vi "calculationView.vi"(11 "View.lvclass":refnum<class "View.lvclass">) -> ()   [LabVIEW 2016, in "View.lvclass"]
uses:
  View.lvclass
  Controller/Controller.lvclass
  Controller/Controller.lvclass/Controller.ctl
  View.lvclass/View.ctl
panel:
  in  "OK Button":bool
  out "Result":dbl
  in  "secondNumber":dbl
  in  "firstNumber":dbl
  # "+"
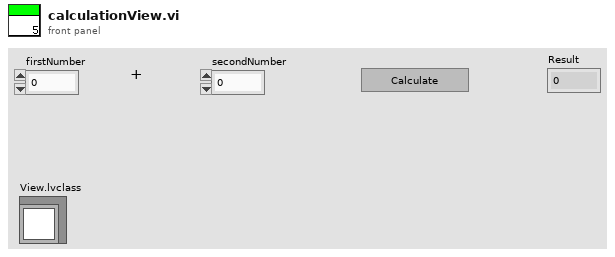
[diagram p1: front panel]
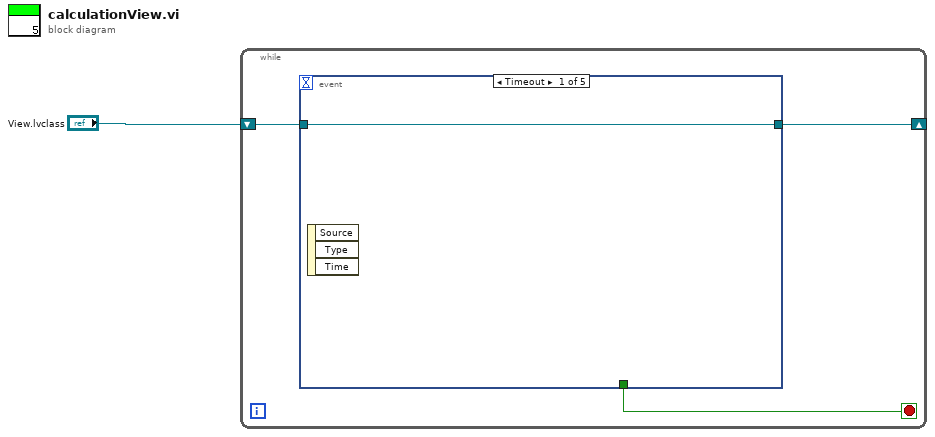
[diagram p0: block diagram]
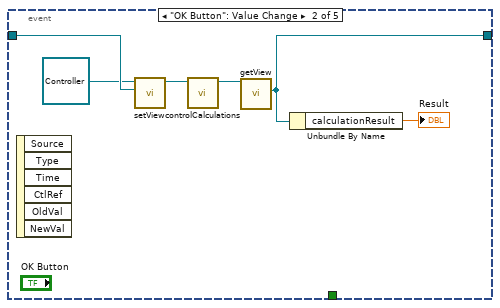
[diagram p2: hidden frame]
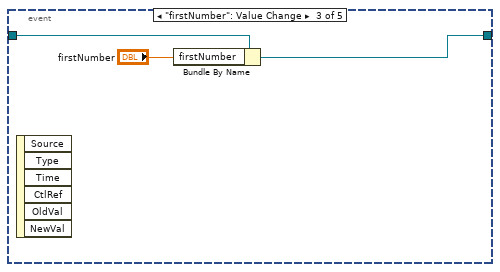
[diagram p3: hidden frame]
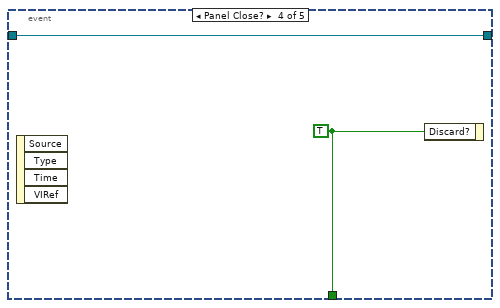
[diagram p4: hidden frame]
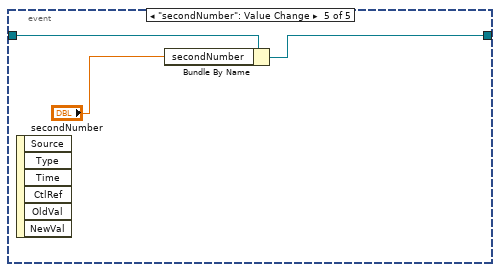
[diagram p5: hidden frame]
diagram:
  n1 = while {
    shift-right: [w2] -> _
    shift-left: "View.lvclass" -> [w4]
    stop <- w3 stop-if-true
    n2 = event shown="[0] Timeout" {
      selector: _ -> [_ _ _ _ _]
      dyn-events: _ -> [_ _ _ _ _]
      timeout: _ -> [_ _ _ _ _]
      tunnel: w4 -> [w5 w10 w14 w15 w18]
      tunnel: [_ _ _ w16 _] -> w3
      tunnel: [w5 w7 w12 w15 w17] -> w2
      event Timeout {
        n3 = event-data() -> ()  [unwired: 1 in, 3 out]
      }
      event "OK Button": Value Change {
        n4 = event-data() -> ()  [unwired: 1 in, 6 out]
        n5 = call "setView.vi"("View.lvclass"=w10, "Controller in"=refnum<class "Controller.lvclass"> refnum) -> ("Controller out"=w11:refnum<class "Controller.lvclass">)  [unwired: 9 in]
        n6 = call "controlCalculations.vi"("Controller In"=w11) -> ("Controller.lvclass"=w9:refnum<class "Controller.lvclass">)  [unwired: 10 in]
        n7 = call "getView.vi"("Controller in"=w9) -> ("View.lvclass"=w7:refnum<class "View.lvclass">)  [unwired: 9 in, 1 out]
        n8 = Unbundle By Name(w7) -> ("calculationResult"=→"Result":dbl)
      }
      event "firstNumber": Value Change {
        n9 = event-data() -> ()  [unwired: 1 in, 6 out]
        n10 = Bundle By Name(cluster=w14, "firstNumber"="firstNumber") -> (w12:refnum<class "View.lvclass">)
      }
      event Panel Close? {
        w16 = TRUE ("Discard?")
        n11 = event-data() -> ()  [unwired: 1 in, 4 out]
        n12 = event-data("Discard?"=w16) -> ()  [unwired: 1 in, 1 out]
      }
      event "secondNumber": Value Change {
        n13 = event-data() -> ()  [unwired: 1 in, 6 out]
        n14 = Bundle By Name(cluster=w18, "secondNumber"="secondNumber") -> (w17:refnum<class "View.lvclass">)
      }
    }
  }
